vi "LogFileWrite.vi"(4 "error in (no error)":errorcluster, 6 "Output Text":string, 7 "CmdLib In":refnum<k24>) -> (0 "error out":errorcluster, 3 "CmdLib Out":refnum<k24>)   [LabVIEW 2013]
uses:
  C:/GEECS/Developers Version/source/Device Driver/Picomotor8742dotNet/NewFocus/CmdLib.dll
  CmdLib.dll
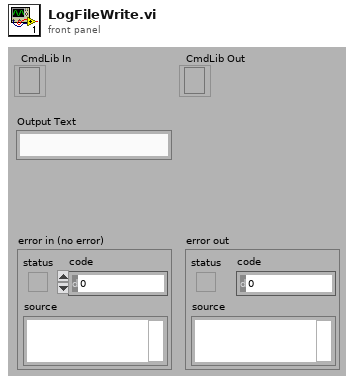
[diagram p1: front panel]
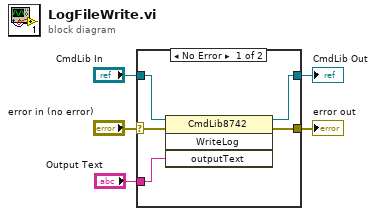
[diagram p0: block diagram]
diagram:
  n1 = case shown="No Error" "error in (no error)" {
    selector: "error in (no error)" -> [w7 w12]
    tunnel: "CmdLib In" -> [w10 w11]
    tunnel: [w9 w11] -> w4
    tunnel: "Output Text" -> [w8 _]
    tunnel: [w6 w12] -> w1
    frame No Error {
      n2 = invoke class="CmdLib8742" method="WriteLog"(reference=w10, error in=w7, "outputText"=w8) -> (reference out=w9:refnum<k24>, error out=w6:errorcluster)  [unwired: 1 in, 2 out]
    }
    frame Error {
    }
  }
  "CmdLib Out" <- w4
  "error out" <- w1
